vi "SMO.Example.TestLauncher.vi"() -> ()   [LabVIEW 2013, in "SMO.Example.lvclass"]
uses:
  SMO.Example.lvclass
  SMO/Typedefs/SMOState --Enum.ctl
  SMO/SMO.lvclass
panel:
  in  "About":bool
  out "error out":errorcluster
  in  "Stop":bool
  # "SMO Test Launcher"
  # "For instructions on how to use the JKI State Machine Objects, examples and video tutorials, visit:\nhttp://jki.net/state-machine-objects/\n\nJKI State Machine Objects™\nhttp://jki.net/state-machine-objects/\nCopyright (C) 2005-2015, JKI <info@jki.net>\nALL RIGHTS RESERVED"
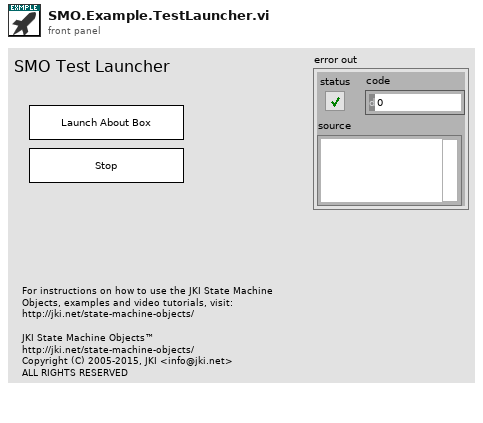
[diagram p1: front panel]
types:
  T1 = typedef "SMO.lvclass/Public Events.ctl" = cluster{"Error":refnum<user-event>, "State":refnum<user-event>}
  T2 = typedef "SMO.Example.lvclass/PublicEvents--Cluster.ctl" = cluster{"Data Changed":refnum<user-event>}
  T3 = typedef "SMO.lvclass/SMOState --Enum.ctl" = enum16{"unknown", "Created", "Started", "Stopped"}
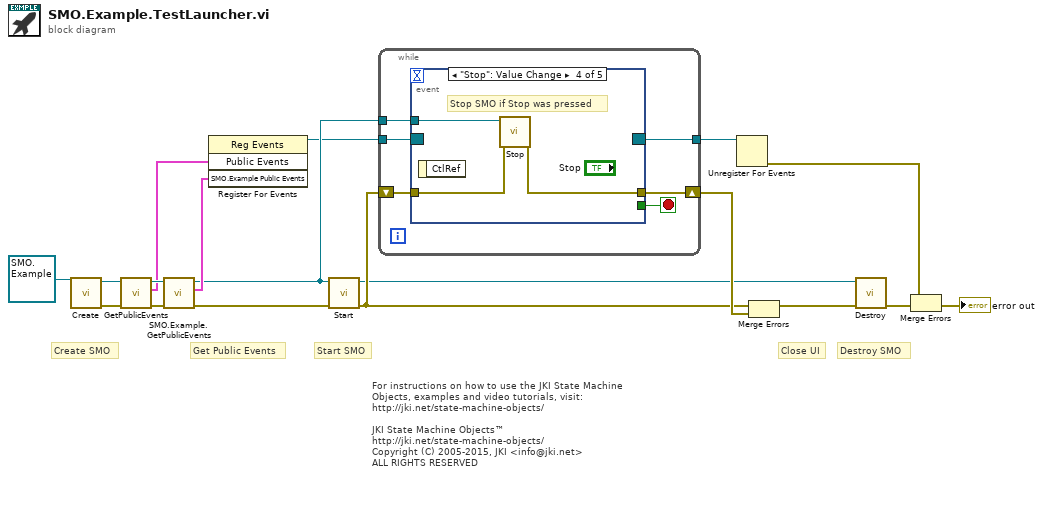
[diagram p0: block diagram]
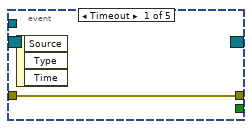
[diagram p2: hidden frame]
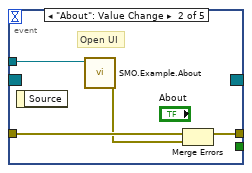
[diagram p3: hidden frame]
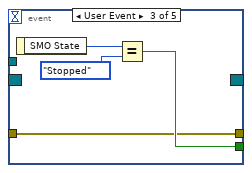
[diagram p4: hidden frame]
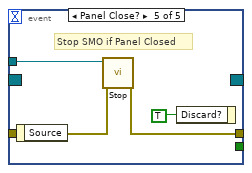
[diagram p5: hidden frame]
diagram:
  # "For instructions on how to use the JKI State Machine Objects, examples and video tutorials, visit:\nhttp://jki.net/state-machine-objects/\n\nJKI State Machine Objects™\nhttp://jki.net/state-machine-objects/\nCopyright (C) 2005-2015, JKI <info@jki.net>\nALL RIGHTS RESERVED"
  # "Get Public Events"
  # "Start SMO"
  # "Destroy SMO"
  # "Create SMO"
  # "Close UI"
  n1 = call "Create.vi"("SMO"=refnum<class "SMO.Example.lvclass"> refnum ("SMO.Example.lvclass")) -> ("error out"=w8:errorcluster, "SMO out"=w9:refnum<class "SMO.Example.lvclass">)  [unwired: 8 in, 1 out]
  n2 = call "GetPublicEvents.vi"("error in (no error)"=w8, "SMO"=w9) -> ("error out"=w7:errorcluster, "Public Events"=w2:T1, "SMO out"=w4:refnum<class "SMO.Example.lvclass">)  [unwired: 7 in]
  n3 = call "SMO.Example.GetPublicEvents.vi"("error in (no error)"=w7, "SMO.Example"=w4) -> ("error out"=w6:errorcluster, "SMO.Example Public Events"=w5:T2, "SMO.Example out"=w3:refnum<class "SMO.Example.lvclass">)  [unwired: 7 in]
  n4 = register-events(w2, w5) -> (reference out=w1:refnum<event-registration>)  [unwired: 2 in, 1 out]
  n5 = call "Start.vi"("error in (no error)"=w6, "SMO"=w3) -> ("error out"=w13:errorcluster, "SMO out"=w12:refnum<class "SMO.Example.lvclass">)  [unwired: 8 in]
  n6 = while {
    shift-right: [w23] -> w17
    shift-left: w13 -> [w22]
    tunnel: w1 -> [w21]
    tunnel: [w20] -> w18
    tunnel: w3 -> [w19]
    stop <- w24 stop-if-true
    n7 = event shown="[3] \"Stop\": Value Change" {
      selector: w21 -> [_ _ _ _ _]
      dyn-events: [_ _ _ _ _] -> w20
      timeout: _ -> [_ _ _ _ _]
      tunnel: [_ _ w31 _ _] -> w24
      tunnel: w19 -> [_ w29 _ w36 w40]
      tunnel: [w25 w26 w30 w35 w39] -> w23
      tunnel: w22 -> [w25 w28 w30 w34 w38]
      event Timeout {
        n8 = event-data() -> ()  [unwired: 1 in, 3 out]
      }
      event "About": Value Change {
        # "Open UI"
        n9 = event-data() -> ()  [unwired: 1 in, 1 out]
        n10 = call "SMO.Example.About.vi"("SMO.Example"=w29) -> ("error out"=w27:errorcluster)  [unwired: 9 in, 1 out]
        n11 = Merge Errors(w28, w27) -> (w26:errorcluster)
      }
      event User Event {
        n12 = event-data() -> ("SMO State"=w33:T3)  [unwired: 1 in]
        n13 = Equal?(x=w33, y=SMOState_--Enum."Stopped") -> (x = y?=w31:bool)
      }
      event "Stop": Value Change {
        # "Stop SMO if Stop was pressed"
        n14 = event-data() -> ()  [unwired: 1 in, 1 out]
        n15 = call "Stop.vi"("error in (no error)"=w34, "SMO"=w36) -> ("error out"=w35:errorcluster)  [unwired: 8 in, 1 out]
      }
      event Panel Close? {
        # "Stop SMO if Panel Closed"
        n16 = event-data() -> ()  [unwired: 1 in, 1 out]
        n17 = call "Stop.vi"("error in (no error)"=w38, "SMO"=w40) -> ("error out"=w39:errorcluster)  [unwired: 8 in, 1 out]
        n18 = event-data("Discard?"=TRUE ("OK")) -> ()  [unwired: 1 in, 1 out]
      }
    }
  }
  n19 = Unregister For Events(event registration refnum=w18) -> (error out=w16:errorcluster)  [unwired: 1 in]
  n20 = Merge Errors(w13, w17) -> (w11:errorcluster)
  n21 = call "Destroy.vi"("error in (no error)"=w11, "SMO"=w12) -> ("error out"=w14:errorcluster)  [unwired: 9 in]
  n22 = Merge Errors(w16, w14) -> (→"error out":errorcluster)
